vi "Is Timing Status Null.vi"(8 "error in (no error)":errorcluster, 11 "timing status pointer in":refnum<class "Timing Status.lvclass">) -> (0 "error out":errorcluster, 2 "null?":bool, 3 "timing status pointer out":refnum<class "Timing Status.lvclass">)   [LabVIEW 2017, in "DSF Core.lvlib" / "Timing Status.lvclass"]
uses:
  Timing Status.lvclass
  C:/Program Files (x86)/National Instruments/LabVIEW 2017/vi.lib/NI/Memory Manager/Classes/Pointer/Pointer.lvclass
  <vilib>/NI/Memory Manager/Classes/Pointer/Pointer.lvclass/Pointer.ctl
  <vilib>/NI/Memory Manager/Classes/Pointer/Get Address.vi
  <vilib>/NI/Memory Manager/Classes/Pointer/Pointer.lvclass
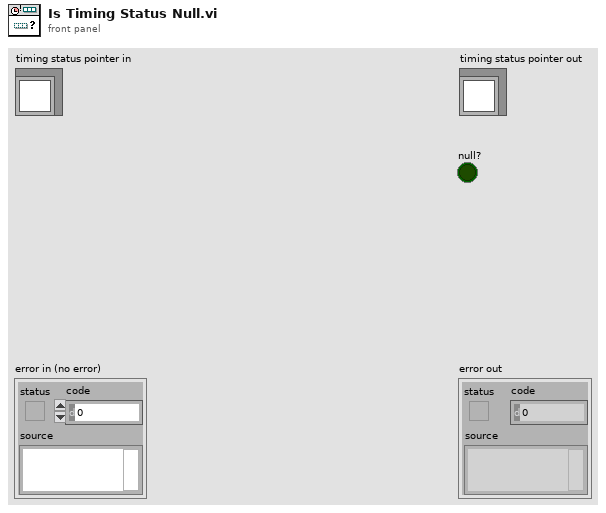
[diagram p1: front panel]
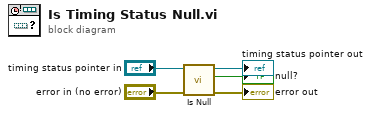
[diagram p0: block diagram]
diagram:
  n1 = call <vilib>:"Is Null.vi"("error in (no error)"="error in (no error)", "Pointer in"="timing status pointer in") -> ("error out"=→"error out":errorcluster, "null?"=→"null?":bool, "Pointer out"=→"timing status pointer out":refnum<class "Timing Status.lvclass">)  [unwired: 7 in]
